vi "ProcessImage.vi"(8 "error in":errorcluster, 11 "Image In":T1 caption="Image Out") -> (0 "error out":errorcluster, 3 "Image Out":T1)   [LabVIEW 2019]
uses:
  <vilib>/vision/Image Controls.llb/IMAQ Image.ctl
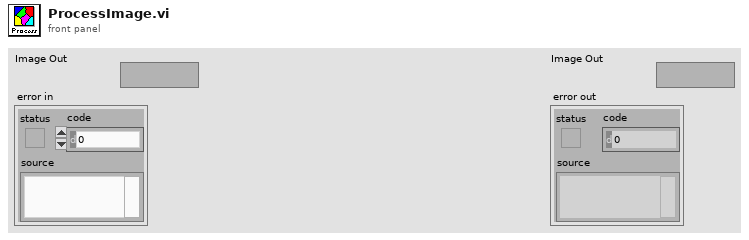
[diagram p1: front panel]
types:
  T1 = typedef "IMAQ Image.ctl" = refnum<image>
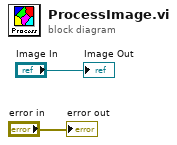
[diagram p0: block diagram]
diagram:
  "Image Out" <- "Image In"
  "error out" <- "error in"
